vi "msd_imp_euler.vi"(0 "M":dbl, 1 "x0":dbl, 2 "v0":dbl, 5 "B":dbl, 7 "K":dbl, 11 "F":dbl, 12 "h":dbl) -> (8 "x1":dbl)   [LabVIEW 2014]
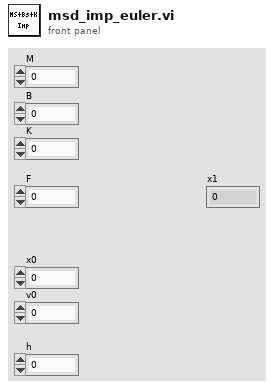
[diagram p1: front panel]
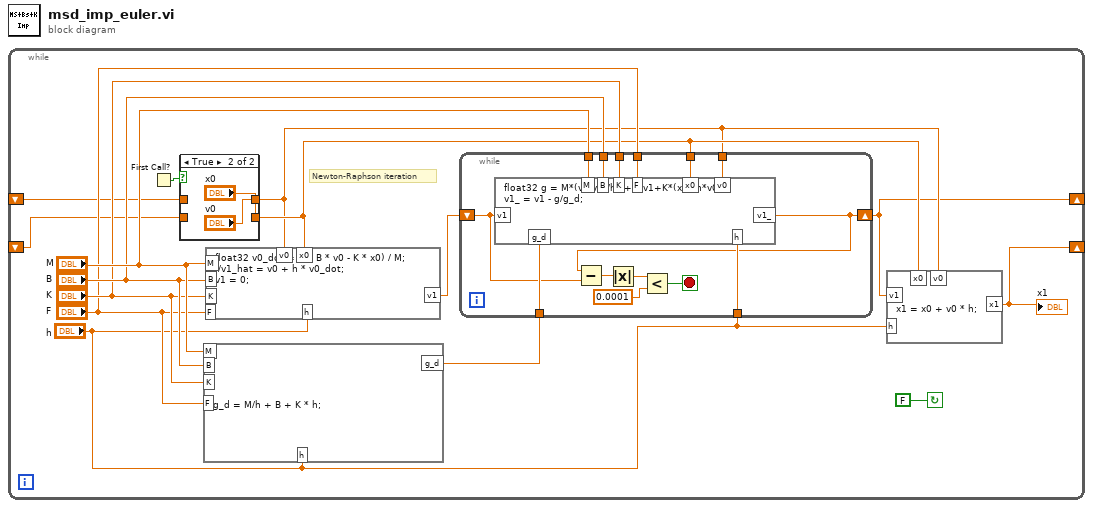
[diagram p0: block diagram]
diagram:
  n1 = while {
    shift-right: [w4] -> _
    shift-left: _ -> [w2]
    shift-right: [w3] -> _
    shift-left: _ -> [w1]
    stop <- FALSE continue-if-true
    # "Newton-Raphson iteration"
    n2 = First Call?() -> (First Call?: T/F=w7:bool)
    n3 = case shown="True" w7 {
      tunnel: [w17 "x0"] -> w6
      tunnel: w2 -> [w17 _]
      tunnel: [w16 "v0"] -> w5
      tunnel: w1 -> [w16 _]
      frame False {
      }
      frame True {
      }
    }
    n4 = formula code="g_d = M/h + B + K * h;"("M"="M", "K"="K", "B"="B", "F"="F", "h"="h") -> ("g_d"=w15:dbl)
    n5 = formula code="float32 v0_dot = (F - B * v0 - K * x0) / M;\n//v1_hat = v0 + h * v0_dot;\nv1 = 0;"("M"="M", "K"="K", "B"="B", "F"="F", "h"="h", "x0"=w6, "v0"=w5) -> ("v1"=w14:dbl)
    n6 = while {
      shift-right: [w20] -> w3
      shift-left: w14 -> [w31]
      tunnel: w15 -> [w33]
      tunnel: "M" -> [w27]
      tunnel: "B" -> [w26]
      tunnel: "K" -> [w25]
      tunnel: "F" -> [w24]
      tunnel: "h" -> [w23]
      tunnel: w6 -> [w22]
      tunnel: w5 -> [w21]
      stop <- w28 stop-if-true
      n7 = formula code="float32 g = M*(v1-v0)/h-F+B*v1+K*(x0+h*v0);\nv1_ = v1 - g/g_d;"("g_d"=w33, "v1"=w31, "M"=w27, "B"=w26, "K"=w25, "F"=w24, "h"=w23, "x0"=w22, "v0"=w21) -> ("v1_"=w20:dbl)
      n8 = Subtract(x=w20, y=w31) -> (x-y=w32:dbl)
      n9 = Absolute Value(x=w32) -> (abs(x)=w30:dbl)
      n10 = Less?(x=w30, y=0.0001) -> (x < y?=w28:bool)
    }
    n11 = formula code="x1 = x0 + v0 * h;"("v1"=w3, "x0"=w6, "v0"=w5, "h"="h") -> ("x1"=w4:dbl)
    "x1" <- w4
  }
